vi "Rad Pin.vi"(7 "Value":bool, 8 "error in (no error)":errorcluster, 9 "Pin":dbl, 10 "Port":dbl, 11 "Module ID":i32=-1) -> (0 "error out":errorcluster)   [LabVIEW 2020, in "Serial Device.lvlib"]
doc: "Evento para poder leer el estado del pin del puerto seleccionado\n_____\nCreated using Delacor QMH Event Scripter 5.0.0.112."
uses:
  Serial Device.lvlib
  Rad Pin Argument--cluster.ctl
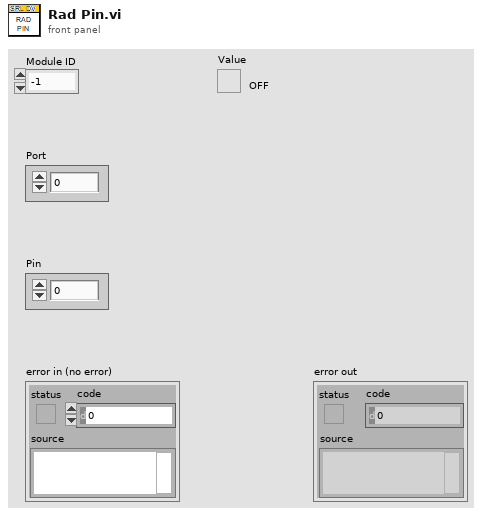
[diagram p1: front panel]
types:
  T1 = typedef "Serial Device.lvlib/Rad Pin Argument--cluster.ctl" = cluster{"Module ID":i32, "Port":dbl, "Pin":dbl, "Value":bool}
  T2 = typedef "Serial Device.lvlib/Request Events--cluster.ctl" = cluster{"Stop Module":refnum<user-event>, "Show Panel":refnum<user-event>, "Hide Panel":refnum<user-event>, "Show Diagram":refnum<user-event>, "Get Module Execution Status":refnum<user-event>, "Write Pin":refnum<user-event>, "Write Port 2":refnum<user-event>, "Read ADC":refnum<user-event>, "Read Port":refnum<user-event>, "Rad Pin":refnum<user-event>}
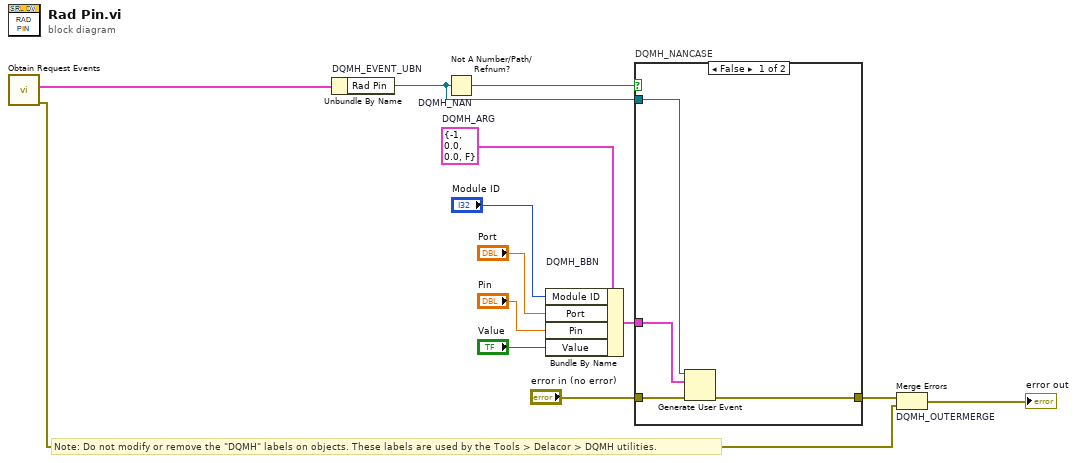
[diagram p0: block diagram]
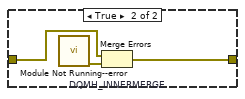
[diagram p2: hidden frame]
diagram:
  w7 = T1 {"Module ID"=-1, "Port"=0.0, "Pin"=0.0, "Value"=FALSE}  # DQMH_ARG
  # "Note: Do not modify or remove the \"DQMH\" labels on objects. These labels are used by the Tools > Delacor > DQMH utilities."
  n1 = call "Obtain Request Events.vi"() -> ("error out"=w2:errorcluster, "Serial Device Request Events"=w1:T2)  [unwired: 10 in]
  n2 = Unbundle By Name "DQMH_EVENT_UBN"(w1) -> ("Rad Pin"=w9:refnum<user-event>)
  n3 = Not A Number/Path/Refnum? "DQMH_NAN"(number/path/refnum=w9) -> (NaN/Path/Refnum?=w10:bool)
  n4 = Bundle By Name "DQMH_BBN"(cluster=w7, "Module ID"="Module ID", "Port"="Port", "Pin"="Pin", "Value"="Value") -> (w11:T1)
  n5 = case "DQMH_NANCASE" shown="False" w10 {
    tunnel: "error in (no error)" -> [w17 w20]
    tunnel: [w16 w19] -> w8
    tunnel: w9 -> [w15 _]
    tunnel: w11 -> [w14 _]
    frame False {
      n6 = Generate User Event(user event=w15, event data cluster=w14, error in=w17) -> (error out=w16:errorcluster)  [unwired: 1 in, 1 out]
    }
    frame True {
      n7 = call "Module Not Running--error.vi"() -> ("error out"=w18:errorcluster)  [unwired: 11 in]
      n8 = Merge Errors "DQMH_INNERMERGE"(w20, w18) -> (w19:errorcluster)
    }
  }
  n9 = Merge Errors "DQMH_OUTERMERGE"(w8, w2) -> (→"error out":errorcluster)
